vi "Legend.vi"() -> ()   [LabVIEW 2013]
uses:
  <vilib>/Heliosphere Research LLC/Advanced Plotting Toolkit/api_annotations/LegendPositions.ctl
  <vilib>/Heliosphere Research LLC/Advanced Plotting Toolkit/api_plotting/LineProperties.ctl
  <vilib>/Heliosphere Research LLC/Advanced Plotting Toolkit/properties/Line.ctl
  <vilib>/Heliosphere Research LLC/Advanced Plotting Toolkit/properties/Line_Style.ctl
  <vilib>/Heliosphere Research LLC/Advanced Plotting Toolkit/typedefs/PlotColor.ctl
  <vilib>/Heliosphere Research LLC/Advanced Plotting Toolkit/properties/Marker.ctl
  <vilib>/Heliosphere Research LLC/Advanced Plotting Toolkit/properties/Marker_Style.ctl
  <vilib>/Heliosphere Research LLC/Advanced Plotting Toolkit/properties/Display.ctl
  <vilib>/Heliosphere Research LLC/Advanced Plotting Toolkit/Advanced Plotting Toolkit.lvlib
panel:
  in  "Legend Position":T1
  in  "Line Title":string="Best Fit"
  in  "Scatter Title":string="Random Data"
  out "Legend Plot":picture
  # "Legend"
  # "Plots made with 1D data, such as those from Line.vi, Scatter.vi,\nBar.vi or Histogram.vi, can have an optional legend labelling\nthe various data sets plotted.\n\nWhen you call such a 1D plotting VI, simply provide the name\nyou would like for the data set.  Then, add a legend to the\nplot by calling Legend.vi.  The populations will be automatically\nlabelled.\n\nData sets plotted with the Legend Title terminal disconnected,\nor with an empty string, do not appear on the legend.  Try\nsetting the \"Scatter Title\" control below to an empty string,\nand see what happens.\n\nFinally, by default the legend will be automatically placed by\nthe Toolkit in an appropriate  place.  You can manually\nspecify the placement to override this; try adjusting the value\nof the \"Legend Position\" control below."
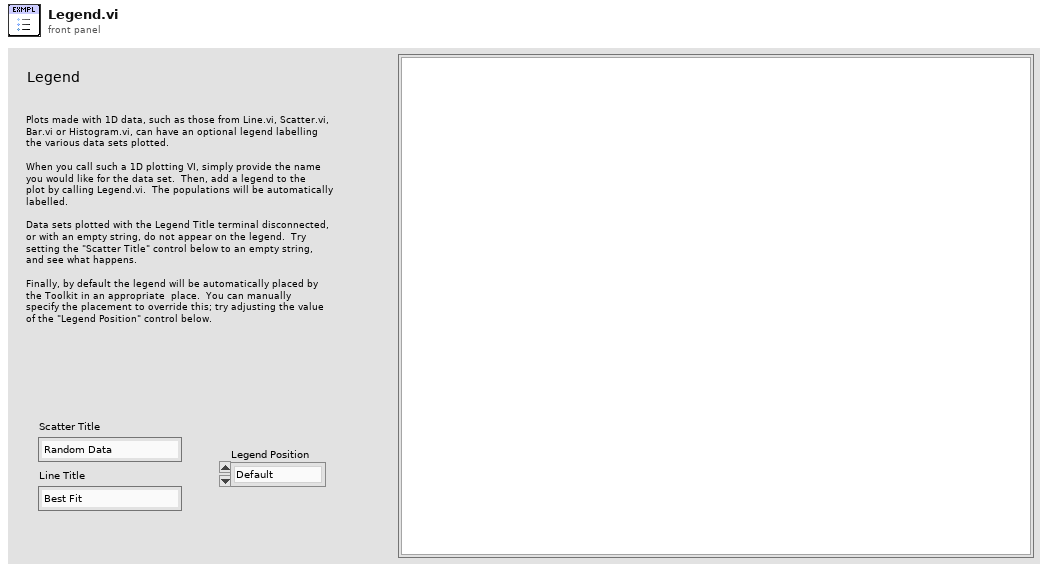
[diagram p1: front panel]
types:
  T1 = typedef "Advanced Plotting Toolkit.lvlib/LegendPositions.ctl" = enum16{"Default", "Top Right", "Top", "Top Left", "Left", "Bottom Left", "Bottom", "Bottom Right", "Right", "Center"}
  T2 = typedef "Advanced Plotting Toolkit.lvlib/Marker_Style.ctl" = enum16{"Automatic", "Circle", "Square", "Triangle", "Diamond", "Star", "Invisible"}
  T3 = typedef "Advanced Plotting Toolkit.lvlib/LineProperties.ctl" = cluster{"Line":T4, "Marker":T7, "Display":T8}
  T4 = typedef "Advanced Plotting Toolkit.lvlib/Line.ctl" = cluster{"Style":T5, "Color":T6, "Width":sgl}
  T5 = typedef "Advanced Plotting Toolkit.lvlib/Line_Style.ctl" = enum16{"Automatic", "Solid", "Dashed", "Dotted", "Dash-dot", "Invisible"}
  T6 = typedef "Advanced Plotting Toolkit.lvlib/PlotColor.ctl" = u32
  T7 = typedef "Advanced Plotting Toolkit.lvlib/Marker.ctl" = cluster{"Style":T2, "Color":T6, "Size":dbl}
  T8 = typedef "Advanced Plotting Toolkit.lvlib/Display.ctl" = cluster{"Alpha":dbl, "Z Order":dbl}
  T9 = typedef "Advanced Plotting Toolkit.lvlib/PlotID.ctl" = i32
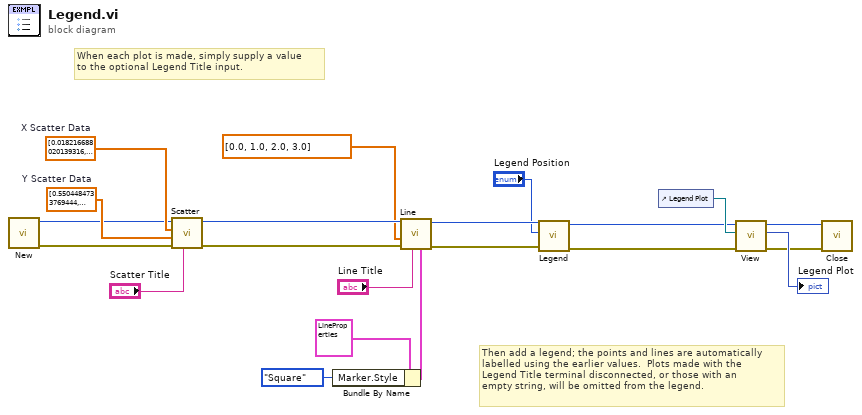
[diagram p0: block diagram]
diagram:
  w17 = dbl[] [0.5504484733769444, 0.7340145289331643, 0.9972841843730318, 0.739103164755676, 0.4719489274133991, 0.48521359909880923, 0.268670749089941, 0.8057782296946243, 0.9028181748401577, 0.7301380893918062, 0.5945088382745651, 0.5664841888262767, 0.6245603532933975, 1.2151753773851341, 1.3751559325201912, 0.7594195233427825, 0.9174437047884547, 0.888032137496148, 1.027309928555396, 0.8465183772390145, 1.4611410254800308, 0.7854320310413877, 1.3305249271114152, 1.4337017682881403, 0.8238392444886502, 1.4695688108297478, 1.5221063546175306, 0.8713493416820589, 1.0954736948939998, 1.6983962844027416, 1.3662143684153685, 1.2125284144057185, 1.1981155398847738, 1.6763550413556394, 1.521911612001944, 1.3177646228410758, 1.413803334048454, 1.639339701921609, 1.6199879794898349, 1.68887714231835, 1.561633324060962, 1.9041851472536078, 1.3852047085256352, 1.7361658644546871, 1.699321108236791, 1.9305833477615097, 1.5819086670974714, 1.7707421705426076, 1.6307798240979468, 1.7271994646006077]  # Y Scatter Data
  w18 = dbl[] [0.018216688020139316, 0.6155646664152035, 0.09161887446563804, 0.5755835424122354, 0.30811405678216486, 0.9300868119887228, 0.7586483780489142, 1.089769759555441, 0.6322835384289796, 0.384787183193845, 1.2778344980742953, 0.9812998154301975, 0.3864217942054192, 1.2257226583790302, 0.5022360656236784, 1.4019622035534751, 0.6452632674815559, 0.8791971175839632, 0.8100268209069452, 1.3321489027970501, 0.6454080555060299, 1.6038888739516306, 0.9794885993611202, 1.201703057246671, 1.3700683222399341, 1.3958110923468907, 1.5420824872003653, 1.5316056401142393, 0.9179293358604258, 1.0770885097208276, 1.0840019398416834, 1.9012209722097482, 1.0103364765183542, 1.4257742799494155, 1.6657001005581127, 1.6988166953387351, 1.6494618253350257, 2.0765624770416053, 2.0856701722269166, 1.4103354500274605, 1.4609448842344637, 2.0763197759765175, 1.6784655640635633, 1.9584138400305964, 2.312762778270861, 1.5973704682789003, 2.0813213329442646, 1.9574908741379595, 2.229063128359036, 1.9824983595019636]  # X Scatter Data
  # "Then add a legend; the points and lines are automatically\nlabelled using the earlier values.  Plots made with the\nLegend Title terminal disconnected, or those with an\nempty string, will be omitted from the legend."
  # "When each plot is made, simply supply a value\nto the optional Legend Title input."
  n1 = call <vilib>:"New.vi"() -> ("error out"=w2:errorcluster, "Plot ID"=w10:T9)  [unwired: 10 in]
  n2 = call <vilib>:"Scatter.vi"("Legend Title"="Scatter Title", "error in (no error)"=w2, "Y Data"=w17, "X Data"=w18, "Plot ID"=w10) -> ("error out"=w15:errorcluster, "Plot ID Out"=w16:T9)  [unwired: 5 in]
  n3 = Bundle By Name(cluster=T3 {"Line"={"Style"=enum."Automatic", "Color"=2147483647, "Width"=nan}, "Marker"={"Style"=enum."Automatic", "Color"=2147483647, "Size"=nan}, "Display"={"Alpha"=nan, "Z Order"=nan}} ("Line Plot Properties"), "Marker.Style"=Marker_Style."Square") -> (w7:T3)
  n4 = call <vilib>:"Line.vi"("Properties"=w7, "Legend Title"="Line Title", "error in (no error)"=w15, "Y Data"=dbl[] [0.0, 1.0, 2.0, 3.0], "Plot ID"=w16) -> ("error out"=w11:errorcluster, "Plot ID out"=w12:T9)  [unwired: 5 in]
  n5 = call <vilib>:"Legend.vi"("error in (no error)"=w11, "Position"="Legend Position", "Plot ID"=w12) -> ("error out"=w13:errorcluster, "Plot ID Out"=w14:T9)  [unwired: 7 in]
  n6 = control-ref of="Legend Plot"() -> (w21:refnum<vi>)
  n7 = call <vilib>:"View.vi"("error in (no error)"=w13, "Ref for Sizing"=w21, "Plot ID"=w14) -> ("error out"=w1:errorcluster, "Picture"=→"Legend Plot":picture, "Plot ID Out"=w19:T9)  [unwired: 6 in]
  n8 = call <vilib>:"Close.vi"("error in (no error)"=w1, "Plot ID"=w19) -> ()  [unwired: 9 in, 1 out]
